vi "Data to 2D String Array.vi"(8 "error in (no error)":errorcluster, 9 "Display Fields":string[](array[combo]), 10 "Query Fields":string[](array[combo]), 11 "Data":variant[][](array[variant])) -> (0 "error out":errorcluster, 3 "data":string[][](array[string]))   [LabVIEW 2021, in "EDT SQLite+.lvlib"]
uses:
  <vilib>/addons/database/_DB Variant To Data/Database Variant To Data.xnode
  EDT SQLite+.lvlib
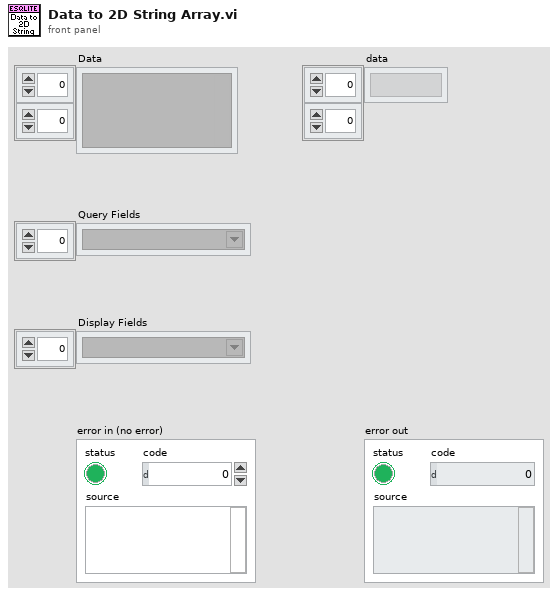
[diagram p1: front panel]
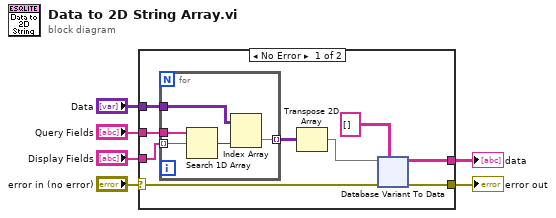
[diagram p0: block diagram]
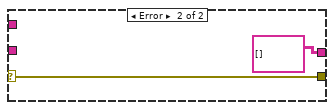
[diagram p2: hidden frame]
diagram:
  n1 = case shown="No Error" "error in (no error)" {
    selector: "error in (no error)" -> [w7 w65]
    tunnel: [w15 string[][] [] ("data")] -> w6
    tunnel: [w14 w65] -> w5
    tunnel: "Data" -> [w10 _]
    tunnel: "Query Fields" -> [w9 _]
    tunnel: "Display Fields" -> [w8 _]
    frame No Error {
      n2 = for {
        tunnel: w8 -> [w63] mode=indexing
        tunnel: w9 -> [w64]
        tunnel: w10 -> [w62]
        tunnel: [w61] -> w11 mode=indexing
        n3 = Search 1D Array(1D array=w64, element=w63) -> (index of element=w60:i32)  [unwired: 1 in]
        n4 = Index Array(array=w62, index (col)=w60) -> (element=w61:variant[])  [unwired: 1 in]
      }
      n5 = Transpose 2D Array(2D array=w11) -> (transposed array=w12:variant[][])
      n6 = xnode "Database Variant To Data"("database variant"=w12, "error in (no error)"=w7, "type"=string[][] []) -> ("data"=w15:string[][], "error out"=w14:errorcluster)
    }
    frame Error {
    }
  }
  "data" <- w6
  "error out" <- w5
